vi "Set MessageQueue.vi"(8 "error in (no error)":errorcluster, 10 "Native Message Queue":refnum<queue>, 11 "MessageQueue in":refnum<class "MessageQueue.lvclass">) -> (0 "error out":errorcluster, 3 "MessageQueue out":refnum<class "MessageQueue.lvclass">)   [LabVIEW 2009, in "LapDog.Messaging.v2.lvlib" / "MessageQueue.lvclass"]
doc: "Accessor method for the native Labview queue refnum. This method is intended for child classes to use when implementing advanced functionality.\n\nThis method ignores all input errors, passing them through unchanged."
uses:
  MessageQueue.lvclass
  MessageObject/Message.lvclass
  MessageQueue.lvclass/MessageQueue.ctl
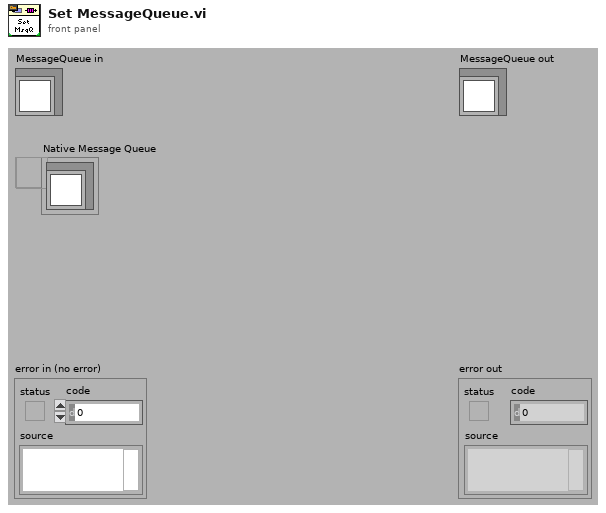
[diagram p1: front panel]
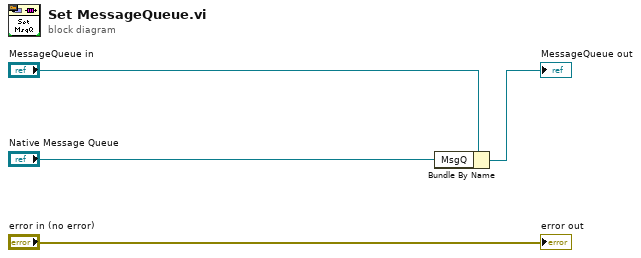
[diagram p0: block diagram]
diagram:
  n1 = Bundle By Name(cluster="MessageQueue in", "MsgQ"="Native Message Queue") -> (→"MessageQueue out":refnum<class "MessageQueue.lvclass">)
  "error out" <- "error in (no error)"
